vi "List Title.vi"(8 "error in (no error)":errorcluster, 11 "List Messages View Model in":refnum<class "List Messages View Model.lvclass">) -> (0 "error out":errorcluster, 2 "Title":string, 3 "List Messages View Model out":refnum<class "List Messages View Model.lvclass">)   [LabVIEW 2020, in "List Messages View Model.lvclass"]
uses:
  List Messages View Model.lvclass
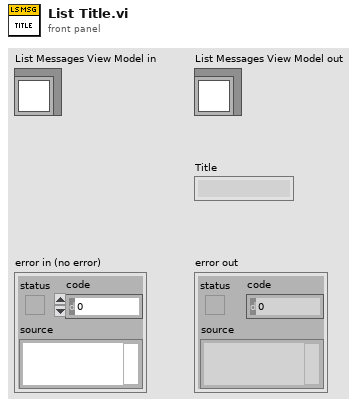
[diagram p1: front panel]
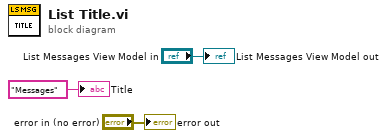
[diagram p0: block diagram]
diagram:
  "error out" <- "error in (no error)"
  "List Messages View Model out" <- "List Messages View Model in"
  "Title" <- "Messages" ("Title")
